vi "Get_Remote_SV_List.vi"(6 "timeout (30 s)":i32=30, 8 "error in (no error)":errorcluster, 11 "Process (\\\\[IPAddress]\\[Process])":string="\\\\127.0.0.1\\System") -> (0 "error out":errorcluster, 3 "Shared Variable List":refnum<k21>[](array[refnum]))   [LabVIEW 2019, in "data.citadel.lvclass"]
doc: "This VI gets a list of Shared Variables on a local or remote process.\n\nCreated By:\nRyan Pacini\n11/31/11"
uses:
  data.citadel.lvclass
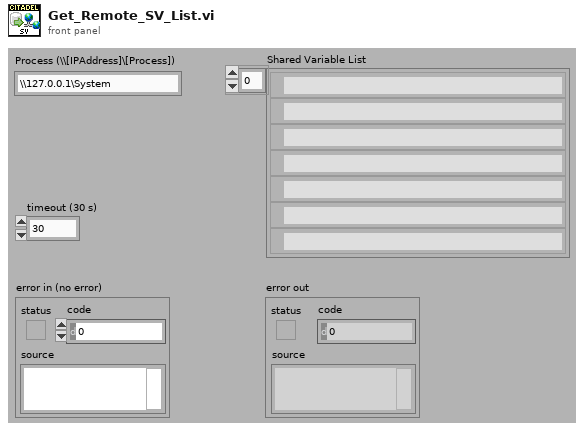
[diagram p1: front panel]
types:
  T1 = enum16{"BT_UNDEFINED", "BT_MACHINE", "BT_PROCESS", "BT_CONTROLENV", "BT_FOLDER", "BT_BLOCK", "BT_BLOCKFOLDER", "BT_ITEM", "BT_ITEMRANGE", "BT_DATABASE", "BT_OPCGROUP", "BT_LKMEMBER", "BT_MEMBER", "BT_CFGOBJECT", "BT_ALARM", "BT_MEMBERRANGE", "BT_LKMEMBERRANGE", "BT_IMPLICIT_MEMBER", "BT_FOLDER_RANGE", "BT_CFGCLASS", "BT_CFGATTR", "BT_NETHOOD", "BT_NETWORK", "BT_DOMAIN", "BT_RUN", "BT_ALARMSERVER"}
  T2 = cluster{"browseType_":enum16{"BT_UNDEFINED", "BT_MACHINE", "BT_PROCESS", "BT_CONTROLENV", "BT_FOLDER", "BT_BLOCK", "BT_BLOCKFOLDER", "BT_ITEM", "BT_ITEMRANGE", "BT_DATABASE", "BT_OPCGROUP", "BT_LKMEMBER", "BT_MEMBER", "BT_CFGOBJECT", "BT_ALARM", "BT_MEMBERRANGE", "BT_LKMEMBERRANGE", "BT_IMPLICIT_MEMBER", "BT_FOLDER_RANGE", "BT_CFGCLASS", "BT_CFGATTR", "BT_NETHOOD", "BT_NETWORK", "BT_DOMAIN", "BT_RUN", "BT_ALARMSERVER"}, "dataType_":u16, "szDelim_":string, "name_":string, "prototype_":variant, "rights_":i16, "BROWSE_FLAGS":u16}[]
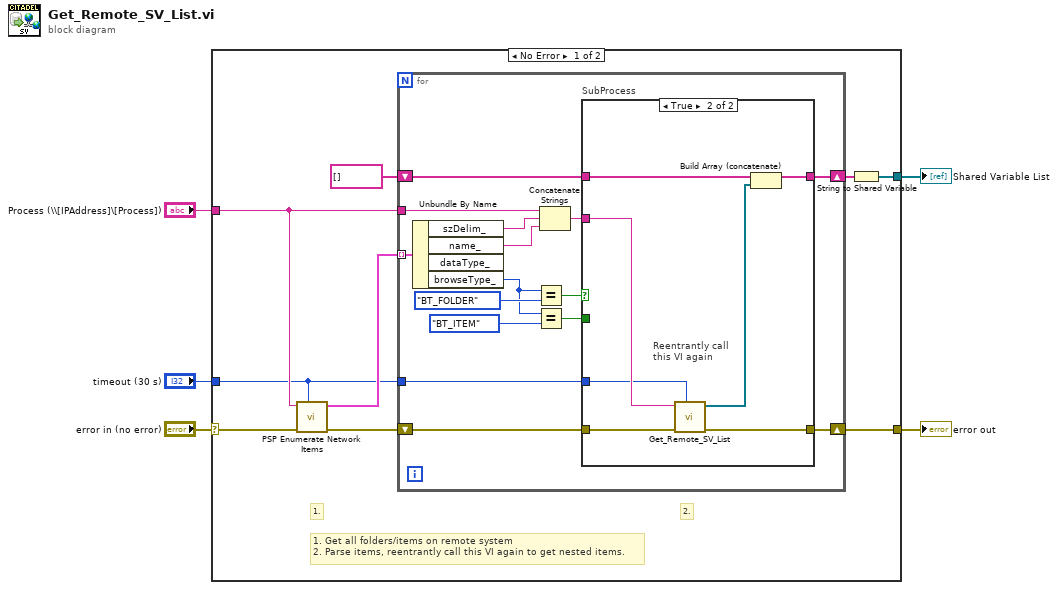
[diagram p0: block diagram]
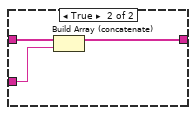
[diagram p3: hidden frame]
diagram:
  n1 = case shown="No Error" "error in (no error)" {
    selector: "error in (no error)" -> [w11 w46]
    tunnel: "Process (\\\\[IPAddress]\\[Process])" -> [w10 _]
    tunnel: [w6 _] -> w4
    tunnel: [w8 w46] -> w3
    tunnel: "timeout (30 s)" -> [w7 _]
    frame No Error {
      # "1. Get all folders/items on remote system\n2. Parse items, reentrantly call this VI again to get nested items."
      # "2."
      # "1."
      n2 = call <vilib>:"PSP Enumerate Network Items.vi"("timeout (30 s)"=w7, "error in (no error)"=w11, "Browse Path"=w10) -> ("error out"=w9:errorcluster, "Items"=w14:T2)  [unwired: 7 in]
      n3 = for {
        tunnel: w14 -> [w27] mode=indexing
        shift-right: [w26] -> w12
        shift-left: string[] [] -> [w25]
        tunnel: w10 -> [w24]
        tunnel: w7 -> [w17]
        shift-right: [w18] -> w8
        shift-left: w9 -> [w19]
        n4 = Unbundle By Name(w27) -> ("szDelim_"=w23:string, "name_"=w22:string, "browseType_"=w15:T1)  [unwired: 1 out]
        n5 = Equal?(x=w15, y=T1."BT_FOLDER" ("browseType_")) -> (x = y?=w28:bool)
        n6 = Equal?(x=w15, y=T1."BT_ITEM" ("browseType_")) -> (x = y?=w16:bool)
        n7 = Concatenate Strings(w24, w23, w22) -> (w21:string)
        n8 = case "SubProcess" shown="True" w28 {
          tunnel: [w31 w40] -> w26
          tunnel: w25 -> [w33 w41]
          tunnel: w21 -> [w32 w43]
          tunnel: w19 -> [w30 w45]
          tunnel: [w30 w44] -> w18
          tunnel: w17 -> [_ w39]
          tunnel: w16 -> [w34 _]
          frame False {
            n9 = case "Variable?" shown="False" w34 {
              tunnel: w33 -> [w35 w38]
              tunnel: w32 -> [_ w36]
              tunnel: [w35 w37] -> w31
              frame False {
                # "Invalid type"
              }
              frame True {
                n10 = Build Array (concatenate)(w38, w36) -> (w37:string[])
              }
            }
          }
          frame True {
            # "Reentrantly call\nthis VI again"
            n11 = call "Get_Remote_SV_List.vi"("timeout (30 s)"=w39, "error in (no error)"=w45, "Process (\\\\[IPAddress]\\[Process])"=w43) -> ("error out"=w44:errorcluster, "Shared Variable List"=w42:refnum<k21>[])  [unwired: 7 in]
            n12 = Build Array (concatenate)(w41, w42) -> (w40:string[])
          }
        }
      }
      n13 = String to Shared Variable(0:w12) -> (2:w6:refnum<k21>[])  [unwired: 1 out]
    }
    frame Error {
    }
  }
  "Shared Variable List" <- w4
  "error out" <- w3
